vi "v1 Elevador.vi"() -> ()   [LabVIEW 2018]
panel:
  in  "Puertas abiertas":bool
  in  "Alarma":bool
  out "Puerta abierta":bool
  in  "PB":bool
  in  "1":bool
  in  "2":bool
  in  "Llamar elevador_PB":bool
  in  "Llamar elevador_1":bool
  in  "Llamar elevador_2":bool
  out "Baja":bool
  out "Sube":bool
  out "Planta Baja":bool
  out "Piso 1":bool
  out "Piso 2":bool
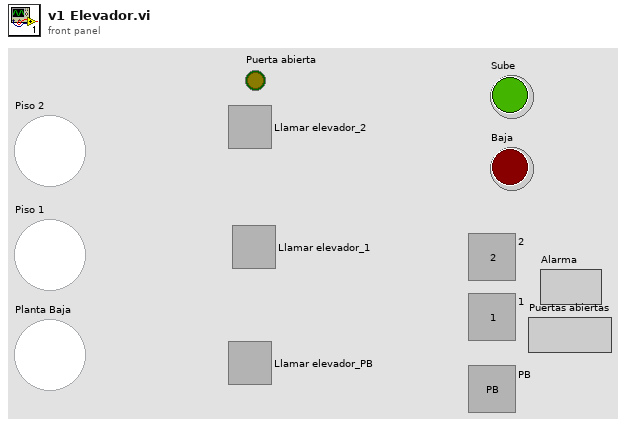
[diagram p1: front panel]
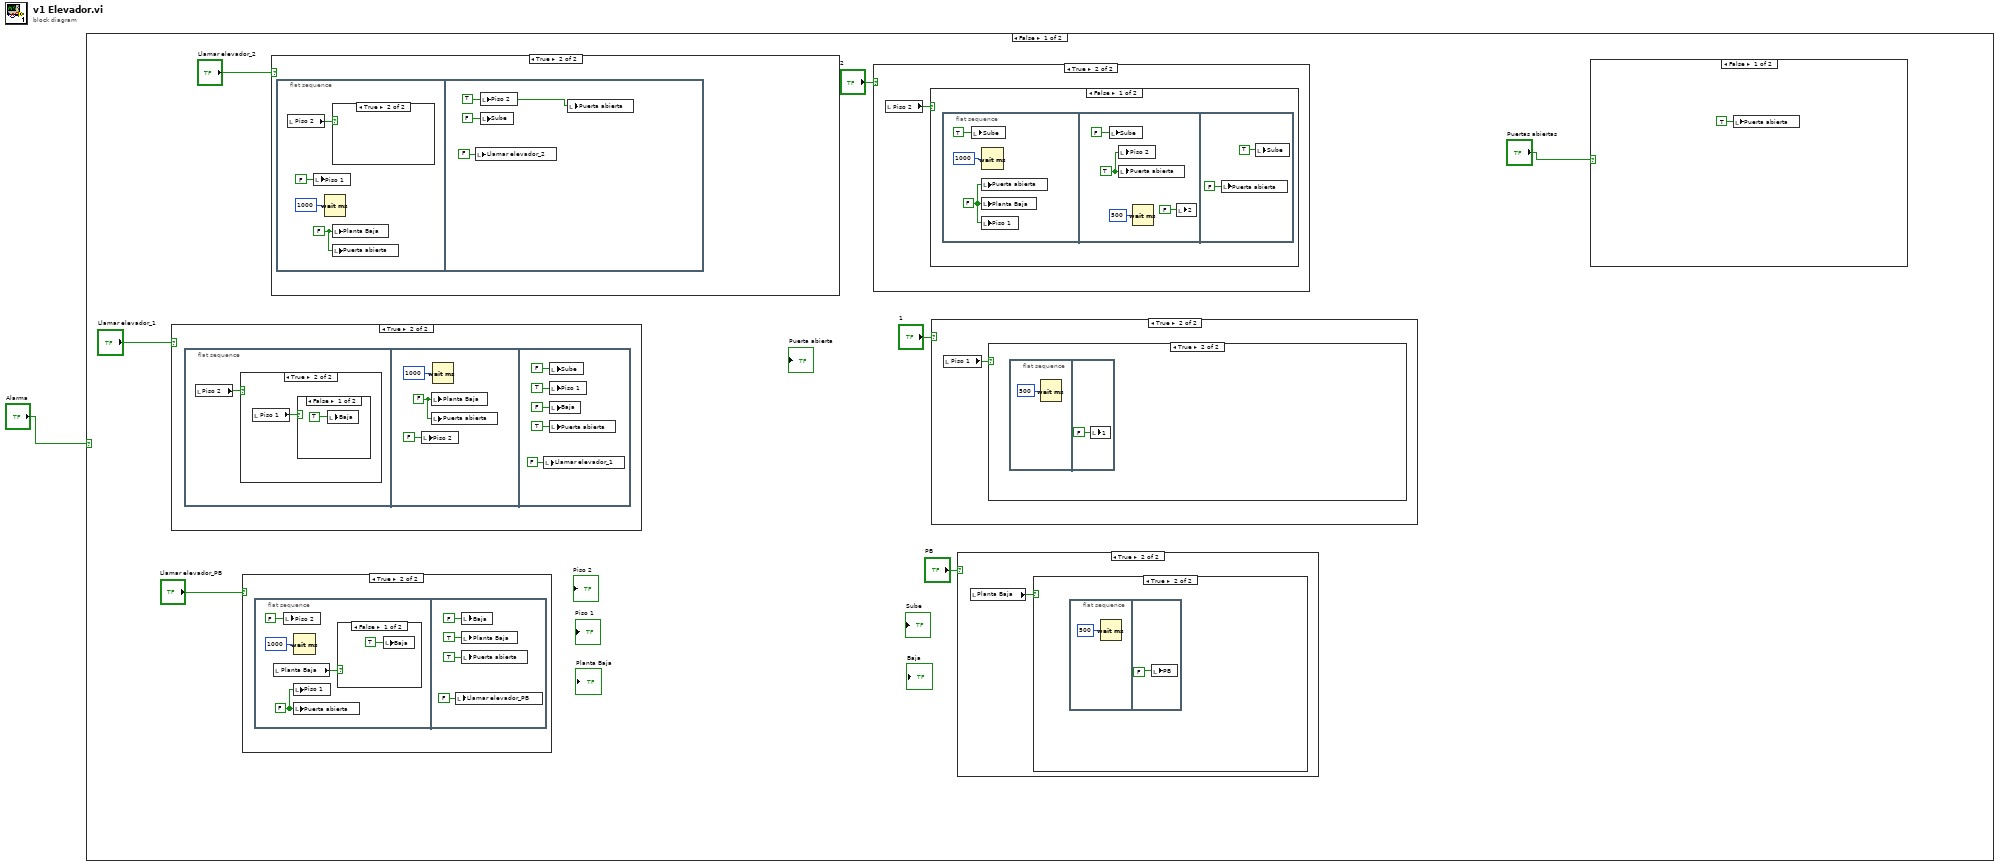
[diagram p0: block diagram]
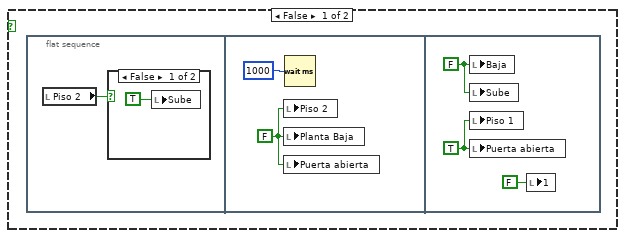
[diagram p4: hidden frame]
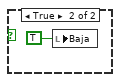
[diagram p5: hidden frame]
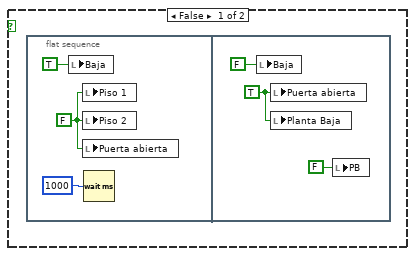
[diagram p7: hidden frame]
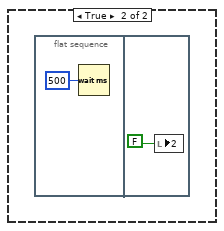
[diagram p9: hidden frame]
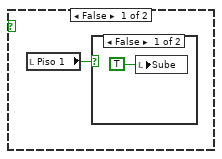
[diagram p13: hidden frame]
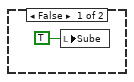
[diagram p17: hidden frame]
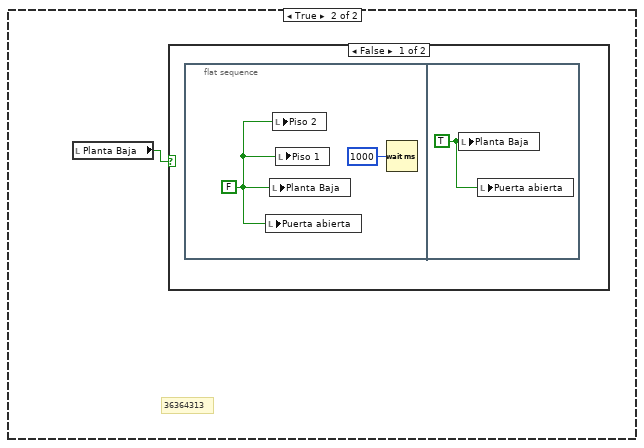
[diagram p18: hidden frame]
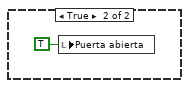
[diagram p19: hidden frame]
diagram:
  n1 = case shown="False" "Alarma" {
    frame False {
      n2 = case shown="True" "Llamar elevador_1" {
        frame False {
        }
        frame True {
          n3 = flat-sequence {
            frame #0 {
              n4 = local read "Piso 2"() -> (w51:bool)
              n5 = case shown="True" w51 {
                frame False {
                  n6 = local read "Piso 1"() -> (w52:bool)
                  n7 = case shown="False" w52 {
                    frame False {
                      n8 = local write "Sube"(TRUE ("Planta Baja")) -> ()
                    }
                    frame True {
                    }
                  }
                }
                frame True {
                  n9 = local read "Piso 1"() -> (w54:bool)
                  n10 = case shown="False" w54 {
                    frame False {
                      n11 = local write "Baja"(TRUE ("Baja")) -> ()
                    }
                    frame True {
                    }
                  }
                }
              }
            }
            frame #1 {
              w56 = FALSE ("Planta Baja")
              n12 = local write "Piso 2"(FALSE ("Piso 2")) -> ()
              n13 = local write "Planta Baja"(w56) -> ()
              n14 = local write "Puerta abierta"(w56) -> ()
              n15 = Wait (ms)(milliseconds to wait=u32 1000) -> ()  [unwired: 1 out]
            }
            frame #2 {
              n16 = local write "Llamar elevador_1"(FALSE ("Llamar elevador_1")) -> ()
              n17 = local write "Sube"(FALSE ("Sube")) -> ()
              n18 = local write "Piso 1"(TRUE ("Piso 1")) -> ()
              n19 = local write "Baja"(FALSE ("Baja")) -> ()
              n20 = local write "Puerta abierta"(TRUE ("Puerta abierta")) -> ()
            }
          }
        }
      }
      n21 = case shown="True" "Llamar elevador_PB" {
        frame False {
        }
        frame True {
          n22 = flat-sequence {
            frame #0 {
              w42 = FALSE ("Piso 1")
              n23 = local read "Planta Baja"() -> (w43:bool)
              n24 = local write "Piso 2"(FALSE ("Piso 2")) -> ()
              n25 = local write "Piso 1"(w42) -> ()
              n26 = local write "Puerta abierta"(w42) -> ()
              n27 = Wait (ms)(milliseconds to wait=u32 1000) -> ()  [unwired: 1 out]
              n28 = case shown="False" w43 {
                frame False {
                  n29 = local write "Baja"(TRUE ("Baja")) -> ()
                }
                frame True {
                }
              }
            }
            frame #1 {
              n30 = local write "Llamar elevador_PB"(FALSE ("Llamar elevador_PB")) -> ()
              n31 = local write "Baja"(FALSE ("Baja")) -> ()
              n32 = local write "Planta Baja"(TRUE ("Planta Baja")) -> ()
              n33 = local write "Puerta abierta"(TRUE ("Puerta abierta")) -> ()
            }
          }
        }
      }
      n34 = case shown="True" "Llamar elevador_2" {
        frame False {
        }
        frame True {
          n35 = flat-sequence {
            frame #0 {
              w64 = FALSE ("Planta Baja")
              n36 = local read "Piso 2"() -> (w65:bool)
              n37 = local write "Piso 1"(FALSE ("Piso 1")) -> ()
              n38 = Wait (ms)(milliseconds to wait=u32 1000) -> ()  [unwired: 1 out]
              n39 = case shown="True" w65 {
                frame False {
                  n40 = local write "Sube"(TRUE ("Sube")) -> ()
                }
                frame True {
                }
              }
              n41 = local write "Planta Baja"(w64) -> ()
              n42 = local write "Puerta abierta"(w64) -> ()
            }
            frame #1 {
              w70 = TRUE ("Piso 2")
              n43 = local write "Llamar elevador_2"(FALSE ("Llamar elevador_2")) -> ()
              n44 = local write "Piso 2"(w70) -> ()
              n45 = local write "Sube"(FALSE ("Sube")) -> ()
              n46 = local write "Puerta abierta"(w70) -> ()
            }
          }
        }
      }
      n47 = case shown="True" "2" {
        frame False {
        }
        frame True {
          n48 = local read "Piso 2"() -> (w30:bool)
          n49 = case shown="False" w30 {
            frame False {
              n50 = flat-sequence {
                frame #0 {
                  w32 = FALSE ("Puerta abierta")
                  n51 = local write "Sube"(TRUE ("Sube")) -> ()
                  n52 = local write "Puerta abierta"(w32) -> ()
                  n53 = local write "Planta Baja"(w32) -> ()
                  n54 = local write "Piso 1"(w32) -> ()
                  n55 = Wait (ms)(milliseconds to wait=u32 1000) -> ()  [unwired: 1 out]
                }
                frame #1 {
                  w36 = TRUE ("Piso 2")
                  n56 = local write "Sube"(FALSE ("Sube")) -> ()
                  n57 = local write "Piso 2"(w36) -> ()
                  n58 = local write "Puerta abierta"(w36) -> ()
                  n59 = Wait (ms)(milliseconds to wait=u32 500) -> ()  [unwired: 1 out]
                  n60 = local write "2"(FALSE ("2")) -> ()
                }
                frame #2 {
                  n61 = local write "Puerta abierta"(FALSE ("Puerta abierta")) -> ()
                  n62 = local write "Sube"(TRUE ("Sube")) -> ()
                }
              }
            }
            frame True {
              n63 = flat-sequence {
                frame #0 {
                  n64 = Wait (ms)(milliseconds to wait=u32 500) -> ()  [unwired: 1 out]
                }
                frame #1 {
                  n65 = local write "2"(FALSE ("1")) -> ()
                }
              }
            }
          }
        }
      }
      n66 = case shown="True" "1" {
        frame False {
        }
        frame True {
          n67 = local read "Piso 1"() -> (w10:bool)
          n68 = case shown="True" w10 {
            frame False {
              n69 = flat-sequence {
                frame #0 {
                  n70 = local read "Piso 2"() -> (w11:bool)
                  n71 = case shown="False" w11 {
                    frame False {
                      n72 = local write "Sube"(TRUE ("Sube")) -> ()
                    }
                    frame True {
                      n73 = local write "Baja"(TRUE ("Baja")) -> ()
                    }
                  }
                }
                frame #1 {
                  w14 = FALSE ("Piso 2")
                  n74 = local write "Piso 2"(w14) -> ()
                  n75 = local write "Planta Baja"(w14) -> ()
                  n76 = local write "Puerta abierta"(w14) -> ()
                  n77 = Wait (ms)(milliseconds to wait=u32 1000) -> ()  [unwired: 1 out]
                }
                frame #2 {
                  w17 = TRUE ("Puerta abierta")
                  w18 = FALSE ("Baja")
                  n78 = local write "Baja"(w18) -> ()
                  n79 = local write "Sube"(w18) -> ()
                  n80 = local write "Piso 1"(w17) -> ()
                  n81 = local write "Puerta abierta"(w17) -> ()
                  n82 = local write "1"(FALSE ("1")) -> ()
                }
              }
            }
            frame True {
              n83 = flat-sequence {
                frame #0 {
                  n84 = Wait (ms)(milliseconds to wait=u32 500) -> ()  [unwired: 1 out]
                }
                frame #1 {
                  n85 = local write "1"(FALSE ("1")) -> ()
                }
              }
            }
          }
        }
      }
      n86 = case shown="True" "PB" {
        frame False {
        }
        frame True {
          n87 = local read "Planta Baja"() -> (w21:bool)
          n88 = case shown="True" w21 {
            frame False {
              n89 = flat-sequence {
                frame #0 {
                  w23 = FALSE ("Piso 1")
                  n90 = local write "Baja"(TRUE ("Baja")) -> ()
                  n91 = local write "Piso 1"(w23) -> ()
                  n92 = local write "Piso 2"(w23) -> ()
                  n93 = local write "Puerta abierta"(w23) -> ()
                  n94 = Wait (ms)(milliseconds to wait=u32 1000) -> ()  [unwired: 1 out]
                }
                frame #1 {
                  w27 = TRUE ("Planta Baja")
                  n95 = local write "Baja"(FALSE ("Baja")) -> ()
                  n96 = local write "Puerta abierta"(w27) -> ()
                  n97 = local write "Planta Baja"(w27) -> ()
                  n98 = local write "PB"(FALSE ("PB")) -> ()
                }
              }
            }
            frame True {
              n99 = flat-sequence {
                frame #0 {
                  n100 = Wait (ms)(milliseconds to wait=u32 500) -> ()  [unwired: 1 out]
                }
                frame #1 {
                  n101 = local write "PB"(FALSE ("1")) -> ()
                }
              }
            }
          }
        }
      }
      n102 = case shown="False" "Puertas abiertas" {
        frame False {
          n103 = local write "Puerta abierta"(TRUE ("Puerta abierta")) -> ()
        }
        frame True {
        }
      }
    }
    frame True {
      # "36364313"
      n104 = local read "Planta Baja"() -> (w72:bool)
      n105 = case shown="False" w72 {
        frame False {
          n106 = flat-sequence {
            frame #0 {
              w74 = FALSE ("Planta Baja")
              n107 = local write "Puerta abierta"(w74) -> ()
              n108 = local write "Planta Baja"(w74) -> ()
              n109 = local write "Piso 2"(w74) -> ()
              n110 = local write "Piso 1"(w74) -> ()
              n111 = Wait (ms)(milliseconds to wait=u32 1000) -> ()  [unwired: 1 out]
            }
            frame #1 {
              w75 = TRUE ("Planta Baja")
              n112 = local write "Planta Baja"(w75) -> ()
              n113 = local write "Puerta abierta"(w75) -> ()
            }
          }
        }
        frame True {
          n114 = local write "Puerta abierta"(TRUE ("Puerta abierta")) -> ()
        }
      }
    }
  }
